vi "replaceWithItemFromNewLibrary.vi"(6 "SubVI Path":path, 8 "error in (no error)":errorcluster, 9 "SubVI Refnum":refnum<vi>, 10 "Calling VI Reference":refnum<vi>, 11 "VI in":refnum<class "VI.lvclass">) -> (0 "error out":errorcluster, 3 "VI out":refnum<class "VI.lvclass">)   [LabVIEW 2016, in "VI.lvclass"]
uses:
  VI.lvclass
  C:/LSST_TS/SystemSW/ct_tools/ProjectItem/ProjectItem.lvclass
  ProjectItem/ProjectItem.lvclass/ProjectItem.ctl
  ProjectItem/ProjectItem.lvclass
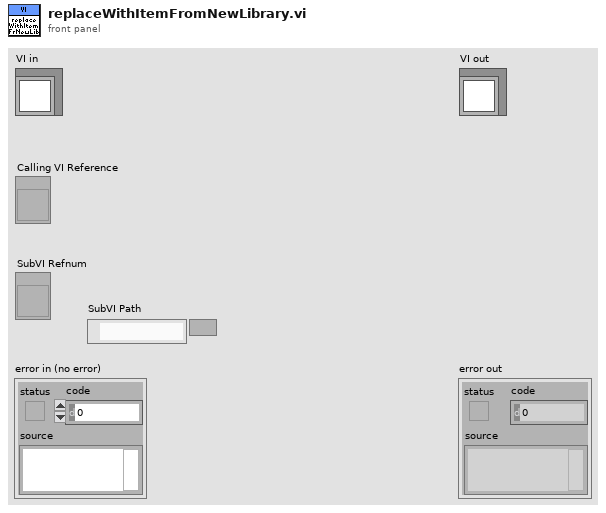
[diagram p1: front panel]
types:
  T1 = typedef "LibraryMemberNameReplacement.ctl" = cluster{"String To Replace in VI names":string, "String To Replace in Control names":string, "New String in VI names":string, "New String in Control names":string}
  T2 = typedef "LibraryDirectories.ctl" = cluster{"OldLibraryDirectory":string, "NewLibraryDirectory":string}
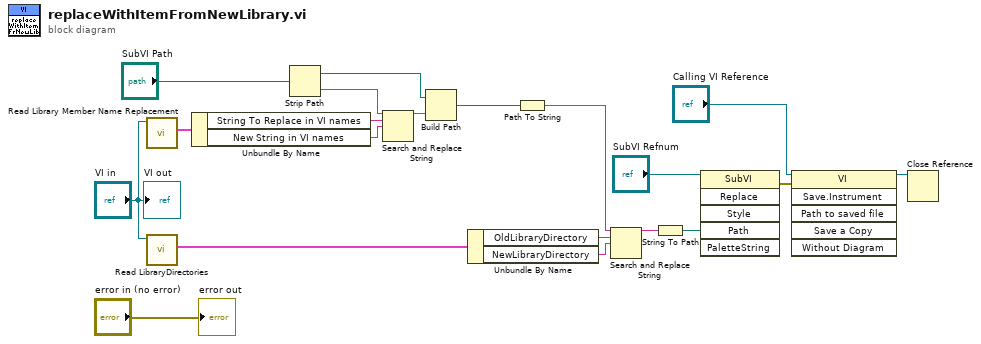
[diagram p0: block diagram]
diagram:
  n1 = call "Read Library Member Name Replacement.vi"("ProjectItem in"="VI in") -> ("Library Member Name Replacement"=w8:T1)  [unwired: 9 in, 1 out]
  n2 = call "Read LibraryDirectories.vi"("ProjectItem in"="VI in") -> ("LibraryDirectories"=w5:T2)  [unwired: 9 in, 1 out]
  n3 = Unbundle By Name(w8) -> ("String To Replace in VI names"=w12:string, "New String in VI names"=w11:string)
  n4 = Strip Path(path="SubVI Path") -> (stripped path=w10:path, name=w13:string)
  n5 = Search and Replace String(input string=w13, search string=w12, replace string=w11) -> (result string=w9:string)  [unwired: 5 in, 3 out]
  n6 = Build Path(base path=w10, name or relative path=w9) -> (appended path=w6:path)
  n7 = Unbundle By Name(w5) -> ("OldLibraryDirectory"=w2:string, "NewLibraryDirectory"=w1:string)
  n8 = Path To String(path=w6) -> (string=w4:string)
  n9 = Search and Replace String(input string=w4, search string=w2, replace string=w1) -> (result string=w3:string)  [unwired: 5 in, 3 out]
  n10 = String To Path(string=w3) -> (path=w18:path)
  n11 = invoke class="SubVI" method="Replace"(reference="SubVI Refnum", "Path"=w18) -> (error out=w16:errorcluster)  [unwired: 4 in, 5 out]
  n12 = invoke class="VI" method="Save.Instrument"(reference="Calling VI Reference", error in=w16) -> (reference out=w19:refnum<vi>)  [unwired: 4 in, 5 out]
  n13 = Close Reference(reference=w19) -> ()  [unwired: 1 in, 1 out]
  "error out" <- "error in (no error)"
  "VI out" <- "VI in"
